vi "Open Motor.vi"(1 "PID?":bool, 2 "Feedback Reference":T1 items=["None"=-1, "QuadEncoder"=0, "Analog"=2, "Tachometer"=4, "Pulse Width Encoded Position"=8, "Sensor Sum (S0 + S1)"=9, "Sensor Difference (D0 - D1)"=10, "Remote Source 0"=11, "Remote Source 1"=12, "Software Emulated"=15], 4 "error in":errorcluster, 5 "refnum name":string="My Motor RefNum", 7 "mode (safety config)":T8, 9 "CAN Device Number":u8, 11 "Set sensor position":dbl, 12 "Reverse Feedback Sensor":bool, 13 "PID gains":T7={"proportional gain (Kc)"=5.0, "integral time (Ti, min)"=0.032, "derivative time (Td, min)"=0.0} {"derivative time (Td, min)" format="%.3f"; "integral time (Ti, min)" format="%.8f"; "proportional gain (Kc)" format="%.8f"}, 14 "Invert Power":bool) -> (6 "CAN Talon SRX Ref":T2={"DeviceStatus"={"status"=FALSE, "code"=0, "source"=""}, "Type"=enum."PWM", "PWM"={"PWM Channel"=enum."PWM 1", "DeadBand"={"Name"="", "maxPositivePwm"=0, "minPositivePwm"=0, "centerPwm"=0, "maxNegativePwm"=0, "minNegativePwm"=0, "angularRange"=0}}, "CAN"={"Device Number"=0, "SetOutput VI Ref"=variant(enum8{"Percent VBus", "Current", "Speed", "Position", "Voltage"} enum."Percent VBus"), "GetOutput VI Ref"=variant(refnum<k1> refnum), "Enable VI Ref"=variant(dbl 12.0), "Disable VI Ref"=variant(enum8{"Percent VBus", "Speed", "Position", "Slave", "Unchanged / Invalid", "Voltage Compensation", "Current", "Motion Profile"} enum."Percent VBus"), "Data"=variant}, "Invert"=FALSE, "DIO PWM"={"PWM \"Enable\" Channel"=enum."Invalid", "DIOChannel"=enum."Invalid", "PWM Rate"=0.0}}, 15 "error out":errorcluster)   [LabVIEW 2017, in "Huskie Swerve.lvlib"]
uses:
  Huskie Swerve.lvlib
  <vilib>/Rock Robotics/WPI/SafetyOutput/WPI_SafetyOutputConfigMenu.ctl
  <vilib>/Rock Robotics/WPI/MotorControl/WPI_MotorControlDeviceRef.ctl
  <vilib>/Rock Robotics/WPI/MotorControl/WPI_MotorControlType.ctl
  <vilib>/Rock Robotics/SystemInterfaces/DIO/FPGA_DIOPWMChannel.ctl
  <vilib>/Rock Robotics/WPI/PWM/WPI_PWMDeadband.ctl
  <vilib>/Rock Robotics/SystemInterfaces/DIO/FPGA_DIOChannel.ctl
  Public/Documents/Cross The Road Electronics/Phoenix-LabVIEW/Motor Controller/Controls/CTRE_Phoenix_MotorControl_FeedbackDevice.ctl
  <vilib>/Rock Robotics/WPI/MotorControl/WPI_MotorControlOpen TalonSRX.vi
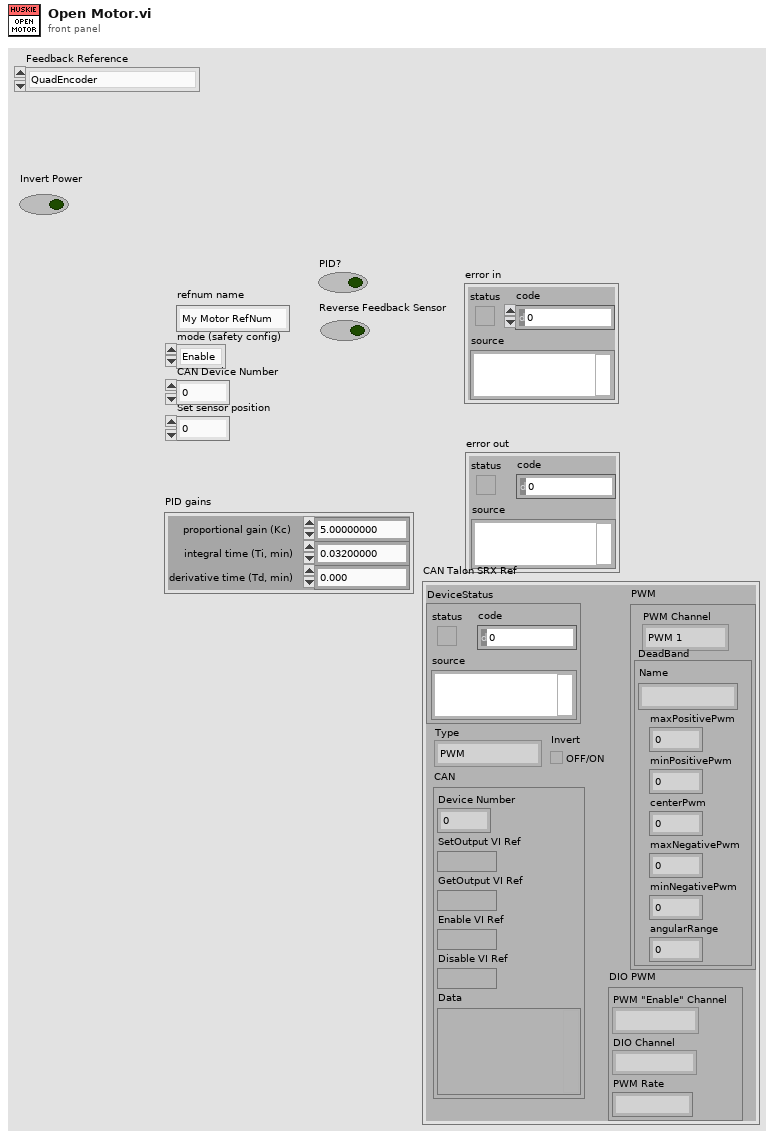
[diagram p1: front panel]
types:
  T1 = typedef "CTRE_Phoenix_MotorControl_FeedbackDevice.ctl" = i8
  T2 = typedef "WPI_MotorControlDeviceRef.ctl" = cluster{"DeviceStatus":errorcluster, "Type":T3, "PWM":cluster{"PWM Channel":T4, "DeadBand":T5}, "CAN":cluster{"Device Number":u8, "SetOutput VI Ref":variant, "GetOutput VI Ref":variant, "Enable VI Ref":variant, "Disable VI Ref":variant, "Data":variant}, "Invert":bool, "DIO PWM":cluster{"PWM \"Enable\" Channel":T4, "DIOChannel":T6, "PWM Rate":dbl}}
  T3 = typedef "WPI_MotorControlType.ctl" = enum16{"PWM", "CAN", "DIO PWM"}
  T4 = typedef "FPGA_DIOPWMChannel.ctl" = enum8{"PWM 0", "PWM 1", "PWM 2", "PWM 3", "PWM 4", "PWM 5", "PWM 6", "PWM 7", "PWM 8", "PWM 9", "PWM MXP 0", "PWM MXP 1", "PWM MXP 2", "PWM MXP 3", "PWM MXP 4", "PWM MXP 5", "PWM MXP 6", "PWM MXP 7", "PWM MXP 8", "PWM MXP 9", "Invalid"}
  T5 = typedef "WPI_PWMDeadband.ctl" = cluster{"Name":string, "maxPositivePwm":i32, "minPositivePwm":i32, "centerPwm":i32, "maxNegativePwm":i32, "minNegativePwm":i32, "angularRange":u16}
  T6 = typedef "FPGA_DIOChannel.ctl" = enum8{"DIO 0", "DIO 1", "DIO 2", "DIO 3", "DIO 4", "DIO 5", "DIO 6", "DIO 7", "DIO 8", "DIO 9", "DIO MXP 0", "DIO MXP 1", "DIO MXP 2", "DIO MXP 3", "DIO MXP 4", "DIO MXP 5", "DIO MXP 6", "DIO MXP 7", "DIO MXP 8", "DIO MXP 9", "DIO MXP 10", "DIO MXP 11", "DIO MXP 12", "DIO MXP 13", "DIO MXP 14", "DIO MXP 15", "SPI Port CS1", "SPI Port CS2", "SPI Port CS3", "SPI Port MISO", "SPI Port MOSI", "Invalid"}
  T7 = cluster{"proportional gain (Kc)":dbl, "integral time (Ti, min)":dbl, "derivative time (Td, min)":dbl}
  T8 = typedef "WPI_SafetyOutputConfigMenu.ctl" = enum16{"Enable", "Disable"}
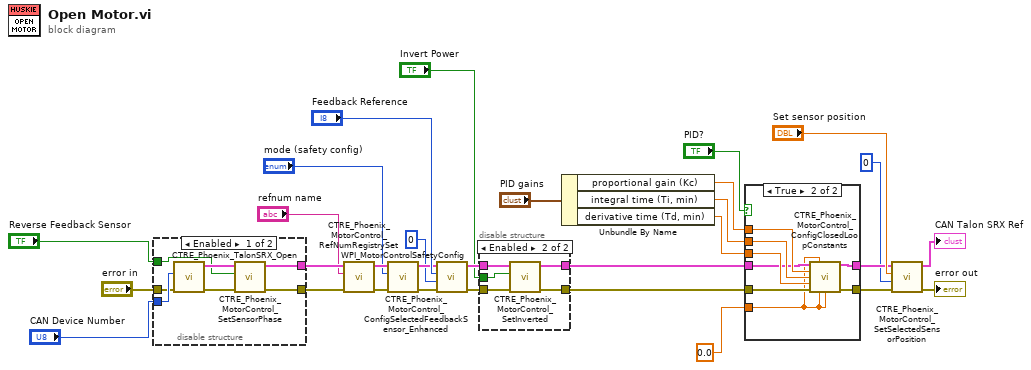
[diagram p0: block diagram]
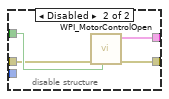
[diagram p2: hidden frame]
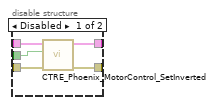
[diagram p3: hidden frame]
diagram:
  n1 = disable-structure shown="Enabled" {
    disable-tunnel: "CAN Device Number" -> [w37 _]
    disable-tunnel: [w32 w38] -> w23
    disable-tunnel: [w35 w39] -> w22
    disable-tunnel: "Reverse Feedback Sensor" -> [w33 w41]
    disable-tunnel: "error in" -> [w36 w40]
    frame Enabled {
      n2 = call "CTRE_Phoenix_TalonSRX_Open.vi"("error in"=w36, "Device Number"=w37) -> ("error out"=w31:errorcluster, "CAN Talon SRX Ref"=w34:T2)  [unwired: 8 in]
      n3 = call "CTRE_Phoenix_MotorControl_SetSensorPhase.vi"("error in (no error)"=w31, "PhaseSensor"=w33, "PhoenixMotorControlDevRef"=w34) -> ("error out"=w32:errorcluster, "PhoenixMotorControlDevRef"=w35:T2)  [unwired: 7 in]
    }
    frame Disabled {
      n4 = call-poly <vilib>:"WPI_MotorControlOpen.vi"("Invert"=w41, "error in (no error)"=w40) -> ("error out"=w38:errorcluster, "MotorControlDeviceRef"=w39:T2)  [unwired: 8 in]
    }
  }
  n5 = call "CTRE_Phoenix_MotorControl_RefNumRegistrySet.vi"("error in (no error)"=w23, "refnum name"="refnum name", "PhoenixMotorControlDevRef"=w22) -> ("error out"=w19:errorcluster, "PhoenixMotorControlDevRef"=w20:T2)  [unwired: 7 in]
  n6 = call <vilib>:"WPI_MotorControlSafetyConfig.vi"("error in (no error)"=w19, "mode"="mode (safety config)", "MotorControlDevRef"=w20) -> ("error out"=w15:errorcluster, "MotorControlDevRef"=w16:T2)  [unwired: 7 in]
  n7 = call "CTRE_Phoenix_MotorControl_ConfigSelectedFeedbackSensor_Enhanced.vi"("error in (no error)"=w15, "pidLoopIdx"=0, "Feedback Device"="Feedback Reference", "PhoenixMotorControlDevRef"=w16) -> ("error out"=w11:errorcluster, "PhoenixMotorControlDevRef"=w14:T2)  [unwired: 6 in]
  n8 = disable-structure shown="Enabled" {
    disable-tunnel: w14 -> [w46 w49]
    disable-tunnel: [w45 w50] -> w13
    disable-tunnel: "Invert Power" -> [w44 w47]
    disable-tunnel: w11 -> [w43 w48]
    disable-tunnel: [w42 w51] -> w10
    frame Disabled {
      n9 = call "CTRE_Phoenix_MotorControl_SetInverted.vi"("error in (no error)"=w43, "Invert?"=w44, "PhoenixMotorControlDevRef"=w46) -> ("error out"=w42:errorcluster, "PhoenixMotorControlDevRef"=w45:T2)  [unwired: 7 in]
    }
    frame Enabled {
      n10 = call "CTRE_Phoenix_MotorControl_SetInverted.vi"("error in (no error)"=w48, "Invert?"=w47, "PhoenixMotorControlDevRef"=w49) -> ("error out"=w51:errorcluster, "PhoenixMotorControlDevRef"=w50:T2)  [unwired: 7 in]
    }
  }
  n11 = Unbundle By Name("PID gains") -> ("proportional gain (Kc)"=w29:dbl, "integral time (Ti, min)"=w28:dbl, "derivative time (Td, min)"=w27:dbl)
  n12 = case shown="True" "PID?" {
    tunnel: w13 -> [w53 w56]
    tunnel: w10 -> [w52 w58]
    tunnel: [w52 w57] -> w5
    tunnel: [w53 w55] -> w8
    tunnel: w29 -> [_ w61]
    tunnel: w28 -> [_ w60]
    tunnel: w27 -> [_ w59]
    tunnel: 0.0 ("New Sensor Position") -> [_ w54]
    frame False {
    }
    frame True {
      n13 = call "CTRE_Phoenix_MotorControl_ConfigClosedLoopConstants.vi"("PhoenixMotorControlDevRef"=w56, "slotIdx"=w54, "P"=w61, "I"=w60, "D"=w59, "error in (no error)"=w58, "F"=w54, "I Zone"=w54) -> ("PhoenixMotorControlDevRef"=w55:T2, "error out"=w57:errorcluster)  [unwired: 6 in]
    }
  }
  n14 = call "CTRE_Phoenix_MotorControl_SetSelectedSensorPosition.vi"("error in (no error)"=w5, "pidLoopIdx"=0, "New Sensor Position"="Set sensor position", "PhoenixMotorControlDevRef"=w8) -> ("error out"=→"error out":errorcluster, "PhoenixMotorControlDevRef"=→"CAN Talon SRX Ref":T2)  [unwired: 6 in]
